vi "sensor_integration.vi"() -> ()   [LabVIEW 2021]
uses:
  <vilib>/Instr/_visa.llb/VISA Configure Serial Port (Instr).vi
  <vilib>/regexp/Match Regular Expression.xnode
panel:
  out "regex error":errorcluster
  out "Array":cluster{dbl, "Numeric":dbl}[](array[cluster]) {"Slide" scale=0.0..20.0}
  out "array":dbl[](array[numeric])
  out "label submatch":string
  out "return count":u32
  in  "stop":bool
  out "read buffer":string
  in  "byte count":u32
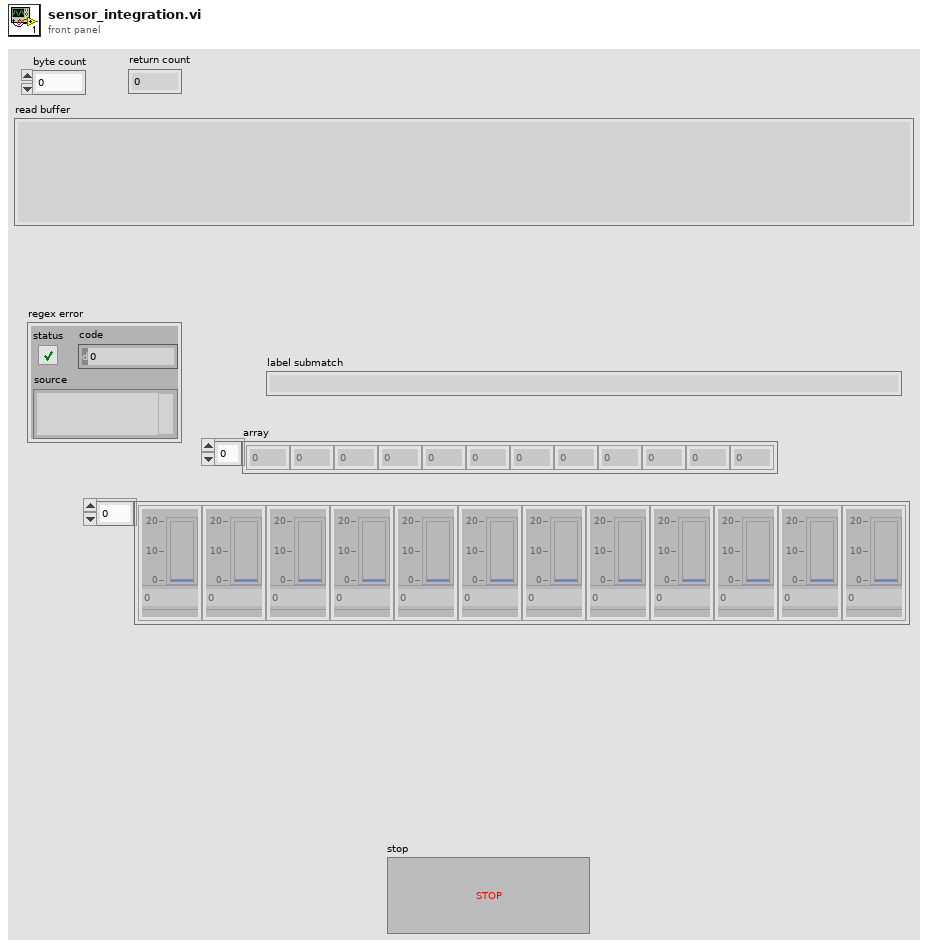
[diagram p1: front panel]
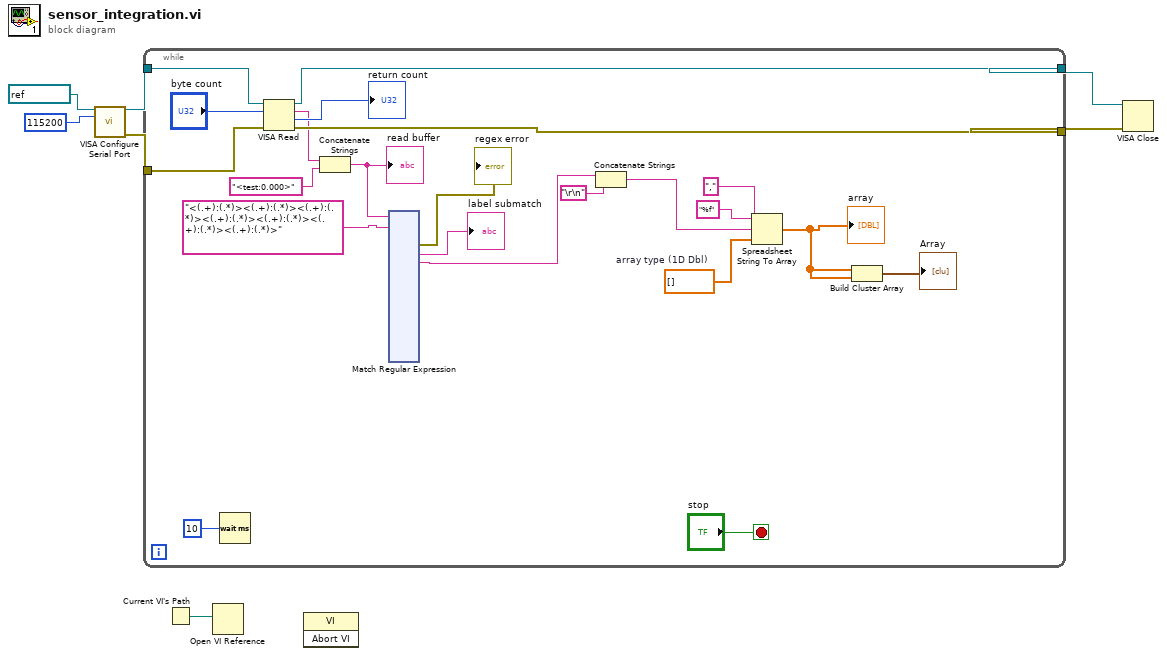
[diagram p0: block diagram]
diagram:
  n1 = call-poly "VISA Configure Serial Port"("VISA resource name"=refnum<visa-resource-name> "COM3", "baud rate (9600)"=u32 115200) -> ("VISA resource name out"=w7:refnum<visa-resource-name>, "error out"=w4:errorcluster)  [unwired: 12 in]
  n2 = while {
    tunnel: w7 -> [w28]
    tunnel: [w26] -> w5
    tunnel: w4 -> [w25]
    tunnel: [w24] -> w3
    stop <- "stop" stop-if-true
    w21 = dbl[] []  # array type (1D Dbl)
    n3 = Wait (ms)(milliseconds to wait=u32 10) -> ()  [unwired: 1 out]
    n4 = VISA Read(VISA resource name=w28, byte count="byte count", error in (no error)=w25) -> (VISA resource name out=w26:refnum<visa-resource-name>, read buffer=w11:string, return count=→"return count":u32, error out=w24:errorcluster)
    n5 = Concatenate Strings(w11, "<test:0.000>" ("string")) -> (w10:string)
    "read buffer" <- w10
    n6 = xnode "Match Regular Expression"("input string"=w10, "regular expression"="<(.+):(.*)><(.+):(.*)><(.+):(.*)><(.+):(.*)><(.+):(.*)><(.+):(.*)><(.+):(.*)>") -> ("error out"=→"regex error":errorcluster, "submatch 1"=→"label submatch":string, "submatch 2"=w8:string)  [unwired: 4 in, 16 out]
    n7 = Concatenate Strings(w8, "\r\n") -> (w17:string)
    n8 = Spreadsheet String To Array(delimiter (Tab)=",", format string="%f", spreadsheet string=w17, array type (2D Dbl)=w21) -> (array=w15:dbl[])
    "array" <- w15
    n9 = Build Cluster Array ("Index & Bundle Cluster Array")(w15, w15) -> (→"Array":cluster{dbl, dbl}[])
  }
  n10 = Current VI's Path() -> (path=w1:path)
  n11 = Open VI Reference(vi path=w1) -> ()  [unwired: 5 in, 2 out]
  n12 = invoke class="VI" method="Abort VI"() -> ()  [unwired: 3 in, 3 out]
  n13 = VISA Close(VISA resource name=w5, error in (no error)=w3) -> ()  [unwired: 1 out]
